vi "TEST.vi"   [LabVIEW 2012]
uses:
  <vilib>/Utility/sysdir.llb/System Directory Type.ctl
  <vilib>/Platform/browser.llb/Open URL in Default Browser (string).vi
types:
  T1 = typedef "System Directory Type.ctl" = i32
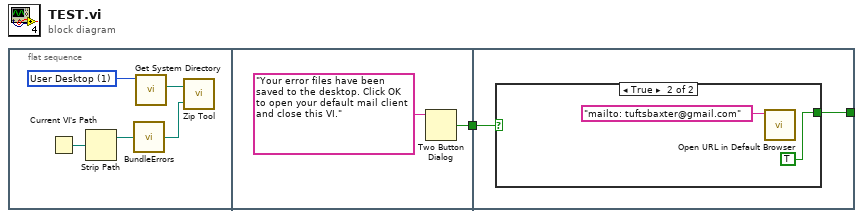
[diagram p0: block diagram]
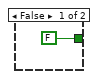
[diagram p2: hidden frame]
diagram:
  n1 = flat-sequence {
    tunnel: [w7] -> w1
    tunnel: w1 -> [w10]
    tunnel: [w9] -> _
    frame #0 {
      w2 = T1 1 items=["User Home"=0, "User Desktop"=1, "User Documents"=2, "User Application Data"=3, "User Preferences"=4, "User Temporary"=5, "Public Documents"=6, "Public Application Data"=7, "Public Preferences"=8, "Public Cache"=13, "System Core Libraries"=9, "System Installed Libraries"=10, "Application Files"=11, "Boot Volume Root"=12] ("system directory type")
      n2 = Current VI's Path() -> (path=w5:path)
      n3 = Strip Path(path=w5) -> (stripped path=w4:path)  [unwired: 1 out]
      n4 = call <userlib>:"BundleErrors.vi"("base path"=w4) -> ("AllErrors"=w6:path)
      n5 = call <vilib>:"Get System Directory.vi"("system directory type"=w2) -> ("system directory"=w3:path)  [unwired: 10 in]
      n6 = call "Zip Tool.vi"("Source File/Directory"=w6, "Target Zip File"=w3) -> ()  [unwired: 1 in]
    }
    frame #1 {
      n7 = Two Button Dialog(message="Your error files have been saved to the desktop. Click OK to open your default mail client and close this VI.") -> (T button?=w7:bool)  [unwired: 2 in]
    }
    frame #2 {
      n8 = case shown="True" w10 {
        tunnel: [FALSE TRUE] -> w9
        frame False {
        }
        frame True {
          n9 = call-poly <vilib>:"Open URL in Default Browser.vi"("URL"="mailto: tuftsbaxter@gmail.com") -> ()  [unwired: 5 in, 2 out]
        }
      }
    }
  }
